vi "Move Straight.vi"(6 "Angle Reduction Factor":dbl, 8 "error in (no error)":errorcluster, 9 "Encoder Reduction Factor":dbl, 10 "Ref-Nums":T1, 11 "Encoder Distance":dbl=-3600.0 format="%#_13g") -> (0 "error out":errorcluster)   [LabVIEW 2016]
uses:
  <vilib>/Rock Robotics/WPI/Utilities/WPI_GetSetVariantRefNum.vi
panel:
  out "Encoder Position":dbl[](graph)
  in  "Reduction Factor 3":dbl
  in  "Encoder Distance 3":dbl=-3600.0 format="%#_13g"
  in  "Reduction Factor 2":dbl
  in  "Encoder Distance 2":dbl=-3600.0 format="%#_13g"
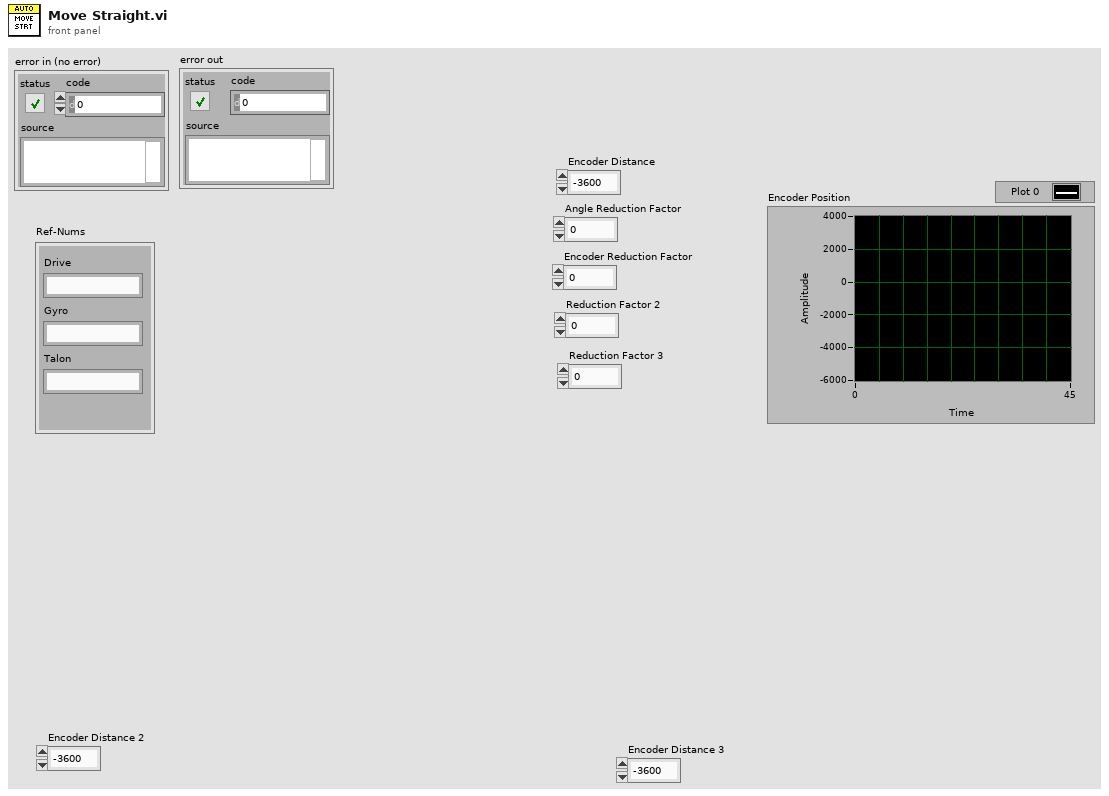
[diagram p1: front panel]
types:
  T1 = cluster{"Drive":string, "Gyro":string, "Talon":string}
  T2 = typedef "WPI_MotorControlDeviceRef.ctl" = cluster{"DeviceStatus":errorcluster, "Type":T3, "PWM":cluster{"PWM Channel":T4, "DeadBand":T5}, "CAN":cluster{"Device Number":u8, "SetOutput VI Ref":variant, "GetOutput VI Ref":variant, "Enable VI Ref":variant, "Disable VI Ref":variant, "Data":variant}, "Invert":bool}
  T3 = typedef "WPI_MotorControlType.ctl" = enum16{"PWM", "CAN"}
  T4 = typedef "FPGA_DIOPWMChannel.ctl" = enum8{"PWM 0", "PWM 1", "PWM 2", "PWM 3", "PWM 4", "PWM 5", "PWM 6", "PWM 7", "PWM 8", "PWM 9", "PWM MXP 0", "PWM MXP 1", "PWM MXP 2", "PWM MXP 3", "PWM MXP 4", "PWM MXP 5", "PWM MXP 6", "PWM MXP 7", "PWM MXP 8", "PWM MXP 9", "Invalid"}
  T5 = typedef "WPI_PWMDeadband.ctl" = cluster{"Name":string, "maxPositivePwm":i32, "minPositivePwm":i32, "centerPwm":i32, "maxNegativePwm":i32, "minNegativePwm":i32, "angularRange":u16}
  T6 = typedef "WPI_CANTalonSRX_GlobalStatus.ctl" = cluster{"Applied Throttle":dbl, "Module Enabled":bool, "CAN Error":errorcluster, "Closed Loop Error":dbl, "Forward Limit Switch Closed":bool, "Reverse Limit Switch Closed":bool, "Sensor Position":dbl, "Sensor Velocity":dbl, "Current":dbl, "Sticky Fault - Over Temp":bool, "Sticky Fault - Under Voltage":bool, "Sticky Fault - Forward Limit":bool, "Sticky Fault - Reverse Limit":bool, "Sticky Fault - Forward Soft Limit":bool, "Sticky Fault - Reverse Soft Limit":bool, "Brake is Enabled":bool, "Encoder Position":dbl, "Encoder Velocity":dbl, "Encoder Index Count":dbl, "Encoder A Pin State":bool, "Encoder B Pin State":bool, "Encoder Index Pin State":bool, "Analog In":dbl, "Analog In Velocity":dbl, "Temperature (C)":dbl, "Battery Voltage":dbl, "Control 5 Is Supported":bool, "Current Profile Slot Select":dbl, "Pos Div 8":bool, "Vel Div 4":bool, "Pulse Width Position":i32, "Pulse Width Velocity":i32, "Pulse Width Rise To Rise (us)":i32, "Pulse Width Rise To Fall (us)":i32, "Mot Prof Active Is Under Run":bool, "Mot Prof Active Has Under Run":bool, "Mot Prof Active Is Last":bool, "Mot Prof Active Velocity Only":bool, "Mot Prof Active Is Valid":bool, "Mot Prof Buffer Is Full":bool, "Mot Prof Active Profile Slot Select":i32, "Mot Prof NextID":i32, "Mot Prof Count":i32, "Mot Prof Active Velocity":dbl, "Mot Prof Active Position":dbl, "Mot Prof Output Enable":i32}
  T7 = typedef "WPI_GyroDevRef.ctl" = cluster{"DevStatus":errorcluster, "Analog Channel":T8, "Offset":dbl, "Gain (VoltsPerDegree/Second)":dbl, "Gyro Type":enum16{"Analog", "XRS450"}, "Handle":i32, "SPI Bus":T9, "Device Found":bool, "Sample Rate":dbl, "Calibrate On Open":bool}
  T8 = typedef "FPGA_AIChannel.ctl" = enum8{"AI 0", "AI 1", "AI 2", "AI 3", "AI MXP 0", "AI MXP 1", "AI MXP 2", "AI MXP 3", "Invalid"}
  T9 = typedef "spi_bus.ctl" = enum16{"SPI On-Board, CS0", "SPI On-Board, CS1", "SPI On-Board, CS2", "SPI On-Board, CS3", "SPI MXP", "Invalid"}
  T10 = typedef "WPI_RobotDriveDevRef.ctl" = cluster{"DevStatus":errorcluster, "Motors[]":T2[], "Square Inputs":bool, "Max Output":dbl}
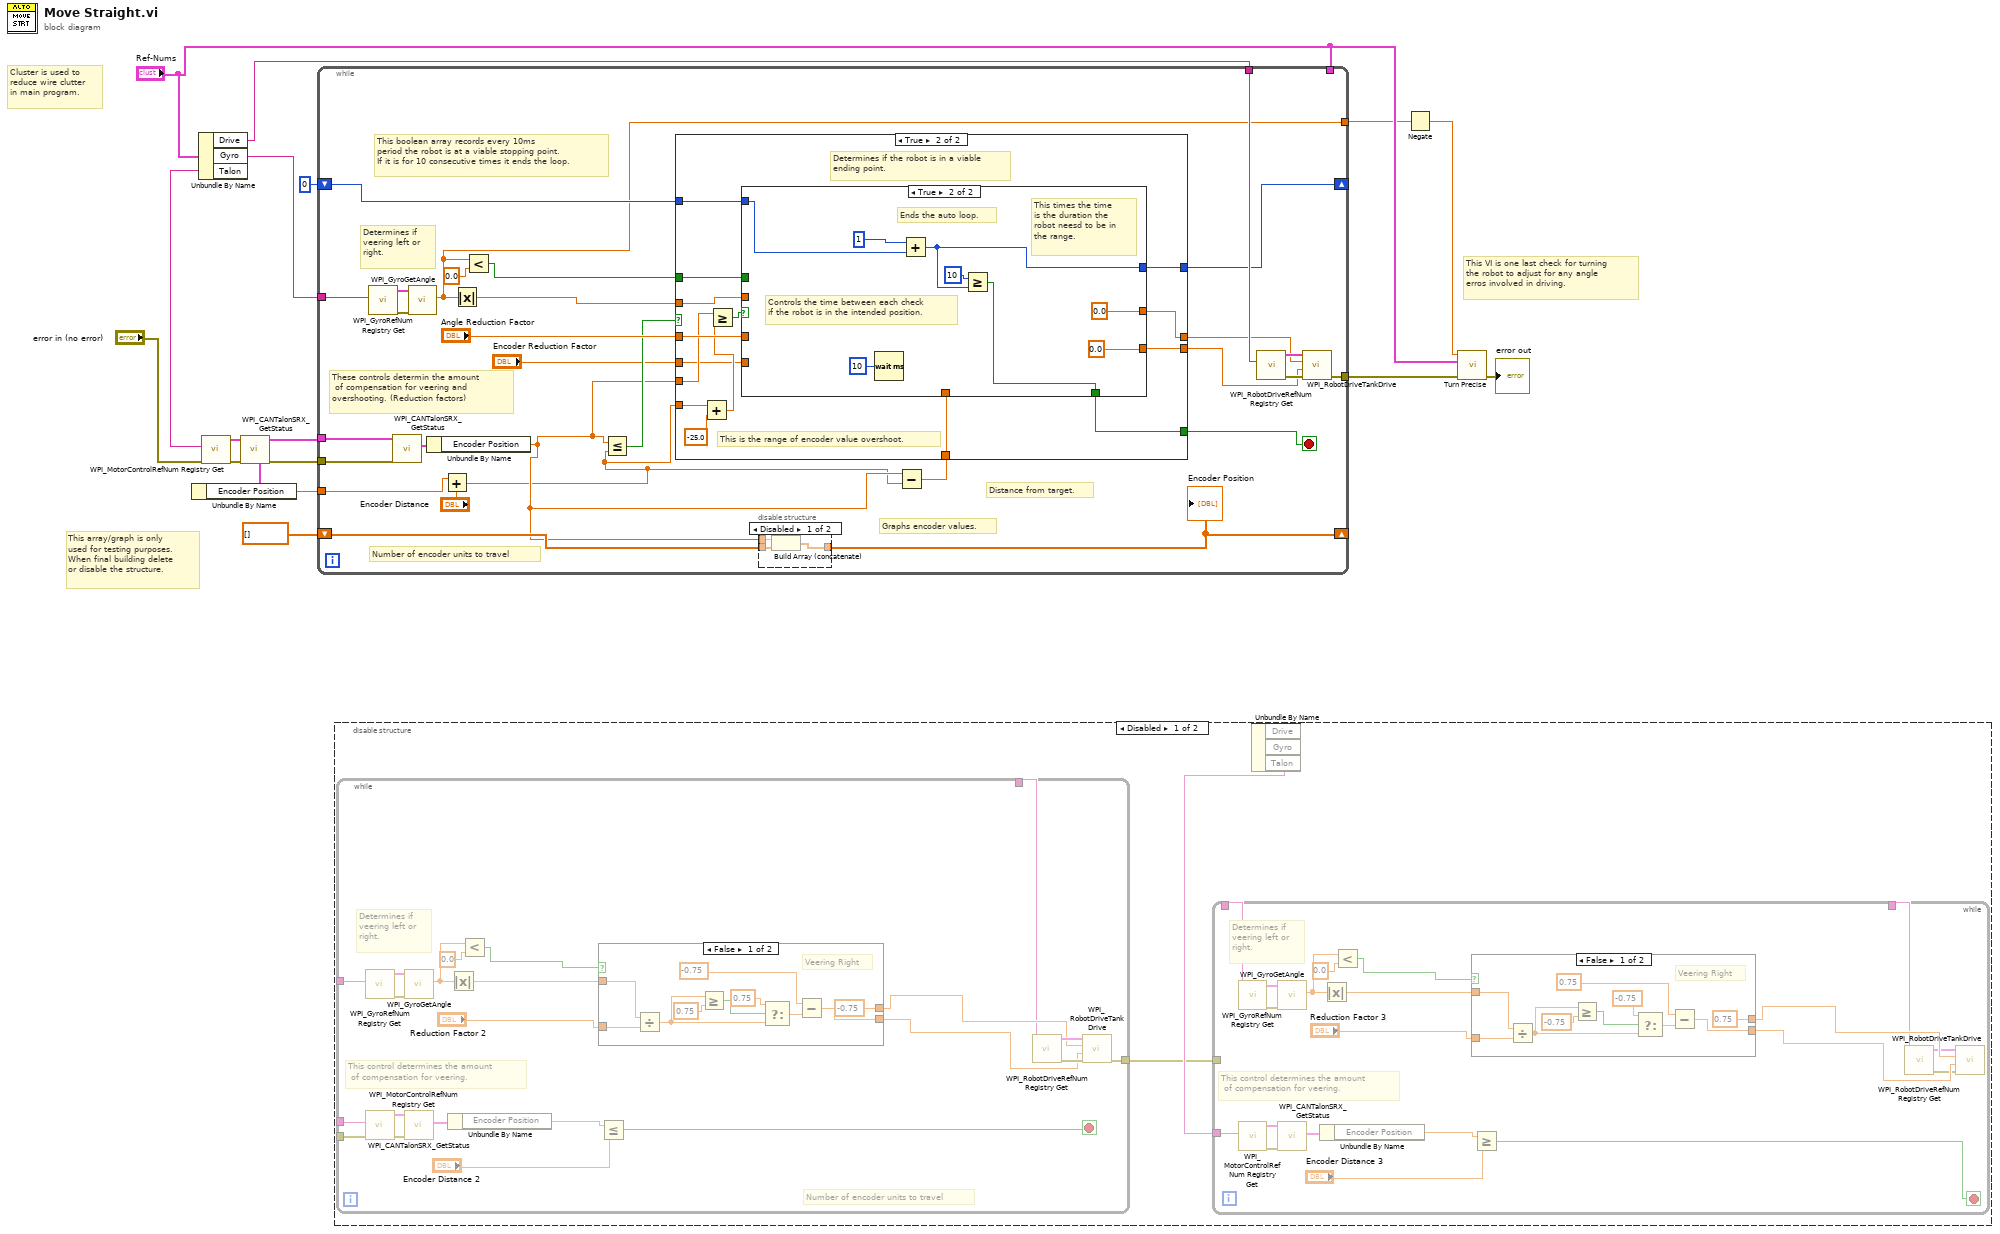
[diagram p0: block diagram]
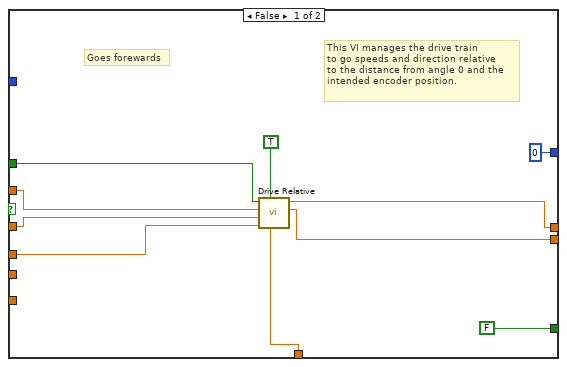
[diagram p3: hidden frame]
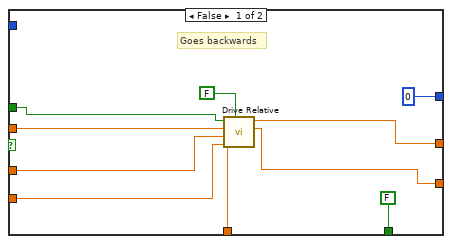
[diagram p4: hidden frame]
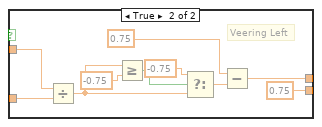
[diagram p5: hidden frame]
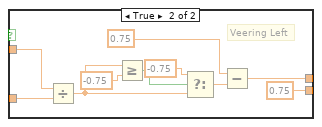
[diagram p6: hidden frame]
diagram:
  # "This VI is one last check for turning\nthe robot to adjust for any angle \nerros involved in driving."
  # "This array/graph is only\nused for testing purposes.\nWhen final building delete\nor disable the structure."
  # "Cluster is used to\nreduce wire clutter\nin main program."
  n1 = Unbundle By Name("Ref-Nums") -> ("Drive"=w16:string, "Gyro"=w17:string, "Talon"=w5:string)
  n2 = call <vilib>:"WPI_MotorControlRefNum Registry Get.vi"("error in (no error)"="error in (no error)", "refnum name"=w5) -> ("error out"=w8:errorcluster, "MotorControlDevRef"=w7:T2)  [unwired: 8 in]
  n3 = call <vilib>:"WPI_CANTalonSRX_GetStatus.vi"("error in (no error)"=w8, "CAN Talon SRX Ref"=w7) -> ("error out"=w2:errorcluster, "Talon SRX Status"=w6:T6, "CAN Talon SRX Ref"=w3:T2)  [unwired: 7 in]
  n4 = Unbundle By Name(w6) -> ("Encoder Position"=w1:dbl)
  n5 = while {
    tunnel: w17 -> [w38]
    tunnel: w3 -> [w24]
    tunnel: w16 -> [w37]
    tunnel: [w36] -> w10
    tunnel: w2 -> [w23]
    shift-right: [w30] -> _
    shift-left: dbl[] [] -> [w31]
    shift-right: [w29] -> _
    shift-left: 0 -> [w28]
    tunnel: [w25] -> w12
    tunnel: "Ref-Nums" -> [_]
    tunnel: w1 -> [w18]
    stop <- w34 stop-if-true
    # "Distance from target."
    # "This boolean array records every 10ms\nperiod the robot is at a viable stopping point.\nIf it is for 10 consecutive times it ends the loop."
    # "Graphs encoder values."
    # "Determines if \nveering left or \nright."
    # "These controls determin the amount\n of compensation for veering and \novershooting. (Reduction factors)"
    # "Number of encoder units to travel"
    n6 = call <vilib>:"WPI_GyroRefNum Registry Get.vi"("refnum name"=w38) -> ("error out"=w41:errorcluster, "GyroDevRef"=w42:T7)  [unwired: 9 in]
    n7 = call <vilib>:"WPI_CANTalonSRX_GetStatus.vi"("error in (no error)"=w23, "CAN Talon SRX Ref"=w24) -> ("Talon SRX Status"=w22:T6)  [unwired: 7 in, 2 out]
    n8 = call <vilib>:"WPI_GyroGetAngle.vi"("error in"=w41, "GyroDevRef"=w42) -> ("Angle"=w25:dbl)  [unwired: 5 in, 4 out]
    n9 = Unbundle By Name(w22) -> ("Encoder Position"=w21:dbl)
    n10 = Add(x=w18, y="Encoder Distance") -> (x+y=w20:dbl)
    n11 = Absolute Value(x=w25) -> (abs(x)=w44:dbl)
    n12 = Less?(x=w25, y=0.0) -> (x < y?=w45:bool)
    n13 = Less Or Equal?(x=w21, y=w20) -> (x <= y?=w35:bool)
    n14 = disable-structure shown="Disabled" {
      disable-tunnel: w31 -> [w49 _]
      disable-tunnel: [w48 _] -> w30
      disable-tunnel: w21 -> [w47 _]
      frame Disabled {
        n15 = Build Array (concatenate)(w47, w49) -> (w48:dbl[])
      }
      frame Enabled {
      }
    }
    "Encoder Position" <- w30
    n16 = Subtract(x=w21, y=w20) -> (x-y=w27:dbl)
    n17 = case shown="True" w35 {
      tunnel: w45 -> [w59 w74]
      tunnel: w44 -> [w58 w73]
      tunnel: "Angle Reduction Factor" -> [w57 w72]
      tunnel: w21 -> [_ w70]
      tunnel: [w56 w66] -> w33
      tunnel: [w55 w65] -> w32
      tunnel: [FALSE w67] -> w34
      tunnel: [0 w64] -> w29
      tunnel: w28 -> [_ w63]
      tunnel: w20 -> [_ w62]
      tunnel: w27 -> [w52 w60]
      tunnel: "Encoder Reduction Factor" -> [w51 w61]
      frame False {
        # "This VI manages the drive train\nto go speeds and direction relative\nto the distance from angle 0 and the\nintended encoder position."
        # "Goes forewards"
        n18 = call "Drive Relative.vi"("Distance From Target"=w52, "Encoder Direction"=TRUE, "Encoder Reduction Factor"=w51, "Angle Reduction Factor"=w57, "Angle"=w58, "Angle Direction"=w59) -> ("Right Power"=w55:dbl, "Left Power"=w56:dbl)  [unwired: 4 in]
      }
      frame True {
        # "This is the range of encoder value overshoot."
        # "Determines if the robot is in a viable\nending point."
        n19 = Add(x=w62, y=-25.0) -> (x+y=w68:dbl)
        n20 = Greater Or Equal?(x=w70, y=w68) -> (x >= y?=w71:bool)
        n21 = case shown="True" w71 {
          tunnel: w74 -> [w82 _]
          tunnel: w73 -> [w81 _]
          tunnel: w72 -> [w80 _]
          tunnel: [FALSE w85] -> w67
          tunnel: [w76 0.0] -> w66
          tunnel: [w77 0.0] -> w65
          tunnel: [0 w87] -> w64
          tunnel: w63 -> [_ w88]
          tunnel: w61 -> [w79 _]
          tunnel: w60 -> [w78 _]
          frame False {
            # "Goes backwards"
            n22 = call "Drive Relative.vi"("Distance From Target"=w78, "Encoder Direction"=FALSE, "Encoder Reduction Factor"=w79, "Angle Reduction Factor"=w80, "Angle"=w81, "Angle Direction"=w82) -> ("Right Power"=w77:dbl, "Left Power"=w76:dbl)  [unwired: 4 in]
          }
          frame True {
            # "This times the time\nis the duration the \nrobot neesd to be in \nthe range."
            # "Controls the time between each check\nif the robot is in the intended position."
            # "Ends the auto loop."
            n23 = Wait (ms)(milliseconds to wait=u32 10) -> ()  [unwired: 1 out]
            n24 = Add(x=1, y=w88) -> (x+y=w87:i32)
            n25 = Greater Or Equal?(x=10, y=w87) -> (x >= y?=w85:bool)
          }
        }
      }
    }
    n26 = call <vilib>:"WPI_RobotDriveRefNum Registry Get.vi"("refnum name"=w37) -> ("error out"=w40:errorcluster, "RobotDriveDevRef"=w39:T10)  [unwired: 9 in]
    n27 = call <vilib>:"WPI_RobotDriveTankDrive.vi"("error in (no error)"=w40, "Right axis value"=w32, "Left axis value"=w33, "RobotDriveDevRef"=w39) -> ("error out"=w36:errorcluster)  [unwired: 5 in, 2 out]
  }
  n28 = disable-structure shown="Disabled" {
    frame Disabled {
      n29 = while {
        tunnel: _ -> [w148]
        tunnel: _ -> [w147]
        tunnel: [w146] -> w93
        tunnel: [w145] -> w95
        tunnel: [w140] -> w94
        stop <- w139 stop-if-true
        # "Determines if \nveering left or \nright."
        # "This control determines the amount\n of compensation for veering."
        # "Number of encoder units to travel"
        n30 = call <vilib>:"WPI_GyroRefNum Registry Get.vi"("refnum name"=w147) -> ("error out"=w155:errorcluster, "GyroDevRef"=w156:T7)  [unwired: 9 in]
        n31 = call <vilib>:"WPI_MotorControlRefNum Registry Get.vi"("error in (no error)"=w148, "refnum name"=w146) -> ("error out"=w149:errorcluster, "MotorControlDevRef"=w150:T2)  [unwired: 8 in]
        n32 = call <vilib>:"WPI_GyroGetAngle.vi"("error in"=w155, "GyroDevRef"=w156) -> ("Angle"=w154:dbl)  [unwired: 5 in, 4 out]
        n33 = call <vilib>:"WPI_CANTalonSRX_GetStatus.vi"("error in (no error)"=w149, "CAN Talon SRX Ref"=w150) -> ("Talon SRX Status"=w151:T6)  [unwired: 7 in, 2 out]
        n34 = Unbundle By Name(w151) -> ("Encoder Position"=w144:dbl)
        n35 = Absolute Value(x=w154) -> (abs(x)=w158:dbl)
        n36 = Less?(x=w154, y=0.0) -> (x < y?=w159:bool)
        n37 = case shown="False" w159 {
          tunnel: [-0.75 w174] -> w142
          tunnel: [w163 0.75] -> w141
          tunnel: w158 -> [w162 w172]
          tunnel: "Reduction Factor 2" -> [w161 w171]
          frame False {
            # "Veering Right"
            n38 = Divide(x=w162, y=w161) -> (x/y=w165:dbl)
            n39 = Greater Or Equal?(x=w165, y=0.75) -> (x >= y?=w169:bool)
            n40 = Select(t=0.75, s=w169, f=w165) -> (s? t:f=w166:dbl)
            n41 = Subtract(x=-0.75 ("y"), y=w166) -> (x-y=w163:dbl)
          }
          frame True {
            # "Veering Left"
            n42 = Divide(x=w172, y=w171) -> (x/y=w175:dbl)
            n43 = Greater Or Equal?(x=w175, y=-0.75) -> (x >= y?=w179:bool)
            n44 = Select(t=-0.75, s=w179, f=w175) -> (s? t:f=w176:dbl)
            n45 = Subtract(x=0.75 ("y"), y=w176) -> (x-y=w174:dbl)
          }
        }
        n46 = Less Or Equal?(x=w144, y="Encoder Distance 2") -> (x <= y?=w139:bool)
        n47 = call <vilib>:"WPI_RobotDriveRefNum Registry Get.vi"("refnum name"=w140) -> ("error out"=w153:errorcluster, "RobotDriveDevRef"=w152:T10)  [unwired: 9 in]
        n48 = call <vilib>:"WPI_RobotDriveTankDrive.vi"("error in (no error)"=w153, "Right axis value"=w141, "Left axis value"=w142, "RobotDriveDevRef"=w152) -> ("error out"=w145:errorcluster)  [unwired: 5 in, 2 out]
      }
      n49 = Unbundle By Name() -> ("Talon"=w98:string)  [unwired: 1 in, 2 out]
      n50 = while {
        tunnel: w95 -> [_]
        tunnel: [w101] -> w96
        tunnel: [w100] -> w97
        tunnel: w98 -> [w99]
        stop <- w102 stop-if-true
        # "Determines if \nveering left or \nright."
        # "This control determines the amount\n of compensation for veering."
        n51 = call <vilib>:"WPI_GyroRefNum Registry Get.vi"("refnum name"=w100) -> ("error out"=w108:errorcluster, "GyroDevRef"=w107:T7)  [unwired: 9 in]
        n52 = call <vilib>:"WPI_MotorControlRefNum Registry Get.vi"("refnum name"=w99) -> ("error out"=w114:errorcluster, "MotorControlDevRef"=w113:T2)  [unwired: 9 in]
        n53 = call <vilib>:"WPI_GyroGetAngle.vi"("error in"=w108, "GyroDevRef"=w107) -> ("Angle"=w109:dbl)  [unwired: 5 in, 4 out]
        n54 = call <vilib>:"WPI_CANTalonSRX_GetStatus.vi"("error in (no error)"=w114, "CAN Talon SRX Ref"=w113) -> ("Talon SRX Status"=w112:T6)  [unwired: 7 in, 2 out]
        n55 = Unbundle By Name(w112) -> ("Encoder Position"=w115:dbl)
        n56 = Absolute Value(x=w109) -> (abs(x)=w105:dbl)
        n57 = Less?(x=w109, y=0.0) -> (x < y?=w104:bool)
        n58 = case shown="False" w104 {
          tunnel: [0.75 w132] -> w117
          tunnel: [w121 0.75] -> w118
          tunnel: w105 -> [w120 w130]
          tunnel: "Reduction Factor 3" -> [w119 w129]
          frame False {
            # "Veering Right"
            n59 = Divide(x=w120, y=w119) -> (x/y=w123:dbl)
            n60 = Greater Or Equal?(x=w123, y=-0.75) -> (x >= y?=w127:bool)
            n61 = Select(t=-0.75, s=w127, f=w123) -> (s? t:f=w124:dbl)
            n62 = Subtract(x=0.75 ("y"), y=w124) -> (x-y=w121:dbl)
          }
          frame True {
            # "Veering Left"
            n63 = Divide(x=w130, y=w129) -> (x/y=w133:dbl)
            n64 = Greater Or Equal?(x=w133, y=-0.75) -> (x >= y?=w137:bool)
            n65 = Select(t=-0.75, s=w137, f=w133) -> (s? t:f=w134:dbl)
            n66 = Subtract(x=0.75 ("y"), y=w134) -> (x-y=w132:dbl)
          }
        }
        n67 = Greater Or Equal?(x=w115, y="Encoder Distance 3") -> (x >= y?=w102:bool)
        n68 = call <vilib>:"WPI_RobotDriveRefNum Registry Get.vi"("refnum name"=w101) -> ("error out"=w110:errorcluster, "RobotDriveDevRef"=w111:T10)  [unwired: 9 in]
        n69 = call <vilib>:"WPI_RobotDriveTankDrive.vi"("error in (no error)"=w110, "Right axis value"=w118, "Left axis value"=w117, "RobotDriveDevRef"=w111) -> ()  [unwired: 5 in, 3 out]
      }
    }
    frame Enabled {
    }
  }
  n70 = Negate(x=w12) -> (-x=w11:dbl)
  n71 = call "Turn Precise.vi"("error in (no error)"=w10, "Ref-Nums"="Ref-Nums", "Angle"=w11) -> ("error out"=→"error out":errorcluster)  [unwired: 8 in]
